vi "RegisterSweepRoutedMessage_Parse.vi"(8 "error in (no error)":errorcluster, 9 "message":variant) -> (0 "error out":errorcluster, 2 "register sweep routed message":T1)   [LabVIEW 2017, in "EmsaDataEventCreator.lvlib"]
uses:
  <vilib>/addons/InsightCM/Devices/Shared/Emsa/EmsaDataEventCreator/EmsaDataEventCreator.lvlib
  <vilib>/addons/InsightCM/Devices/Shared/Emsa/EmsaDataEventCreator/controls/RegisterSweepRoutedMessage.ctl
  <vilib>/addons/InsightCM/Devices/Shared/Emsa/EmsaDataEventCreator/controls/Registry_Sweep.ctl
  <vilib>/addons/InsightCM/Devices/Shared/Common/DataEvent/controls/DataSetType.ctl
  <vilib>/addons/InsightCM/MessageBus/Base/controls/KeyValuePair.ctl
  <vilib>/addons/InsightCM/Devices/Shared/Common/DataEvent/DataEvent.lvlib
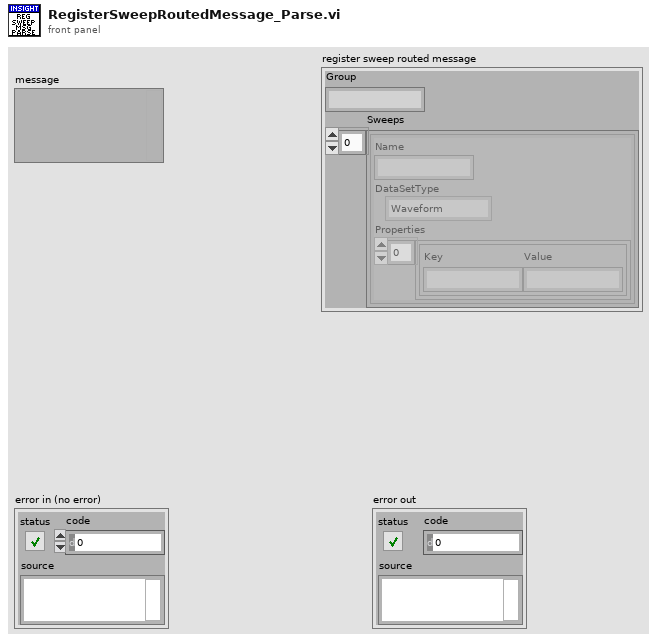
[diagram p1: front panel]
types:
  T1 = typedef "EmsaDataEventCreator.lvlib/RegisterSweepRoutedMessage.ctl" = cluster{"Group":string, "Sweeps":T2[]}
  T2 = typedef "EmsaDataEventCreator.lvlib/Registry_Sweep.ctl" = cluster{"Name":string, "DataSetType":T3, "Properties":T4[]}
  T3 = typedef "DataEvent.lvlib/DataSetType.ctl" = enum16{"Waveform", "SpeedProfile", "ThermalImage", "EmsaSweep"}
  T4 = typedef "KeyValuePair.ctl" = cluster{"Key":string, "Value":string}
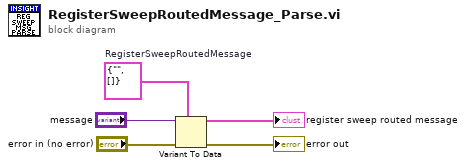
[diagram p0: block diagram]
diagram:
  w2 = T1 {"Group"="", "Sweeps"=[]}  # RegisterSweepRoutedMessage
  n1 = Variant To Data(error in="error in (no error)", type=w2, Variant="message") -> (data=→"register sweep routed message":T1, error out=→"error out":errorcluster)
